vi "6-step.vi"(3 "this":i32, 4 "button":i32, 5 "shift in":bool, 6 "settings in":T1={"Auto1"=TRUE, "Auto2"=TRUE, "Rel1"=TRUE, "Rel2"=TRUE, "Filt1"=TRUE, "Filt2"=TRUE, "Rate"=enum."Slow", "Range1"=enum."10mV", "Range2"=enum."100mV", "Filt3"=TRUE, "Filt4"=TRUE, "Rel temp 1"=TRUE, "Analog1"=FALSE, "Analog2"=FALSE, "Analog temp 1"=FALSE, "Digital1"=TRUE, "Digital2"=TRUE, "Digital temp 1 "=TRUE, "Window1"=enum."0,01%", "Window2"=enum."0,01%", "Window temp 1"=enum."0,01%", "RDGS1"="010", "RDGS2"="010", "RDGS temp 1"="010", "Type_type1"=TRUE, "Type_type2"=TRUE, "Type_type temp 1"=TRUE, "LSync"=FALSE, "Unit"=enum."C", "Sens"=TRUE, "Type tcoupl"=enum."J", "Junc"=TRUE, "prevState"=0, "Rel temp 2"=TRUE, "Analog temp 2"=FALSE, "Digital temp 2"=TRUE, "Type_type temp 2"=TRUE, "RDGS temp 2"="010", "Window temp 2"=enum."0,01%", "addres"="0"}) -> (0 "next state":i32, 1 "shift out":bool, 2 "settings out":T1)   [LabVIEW 2017]
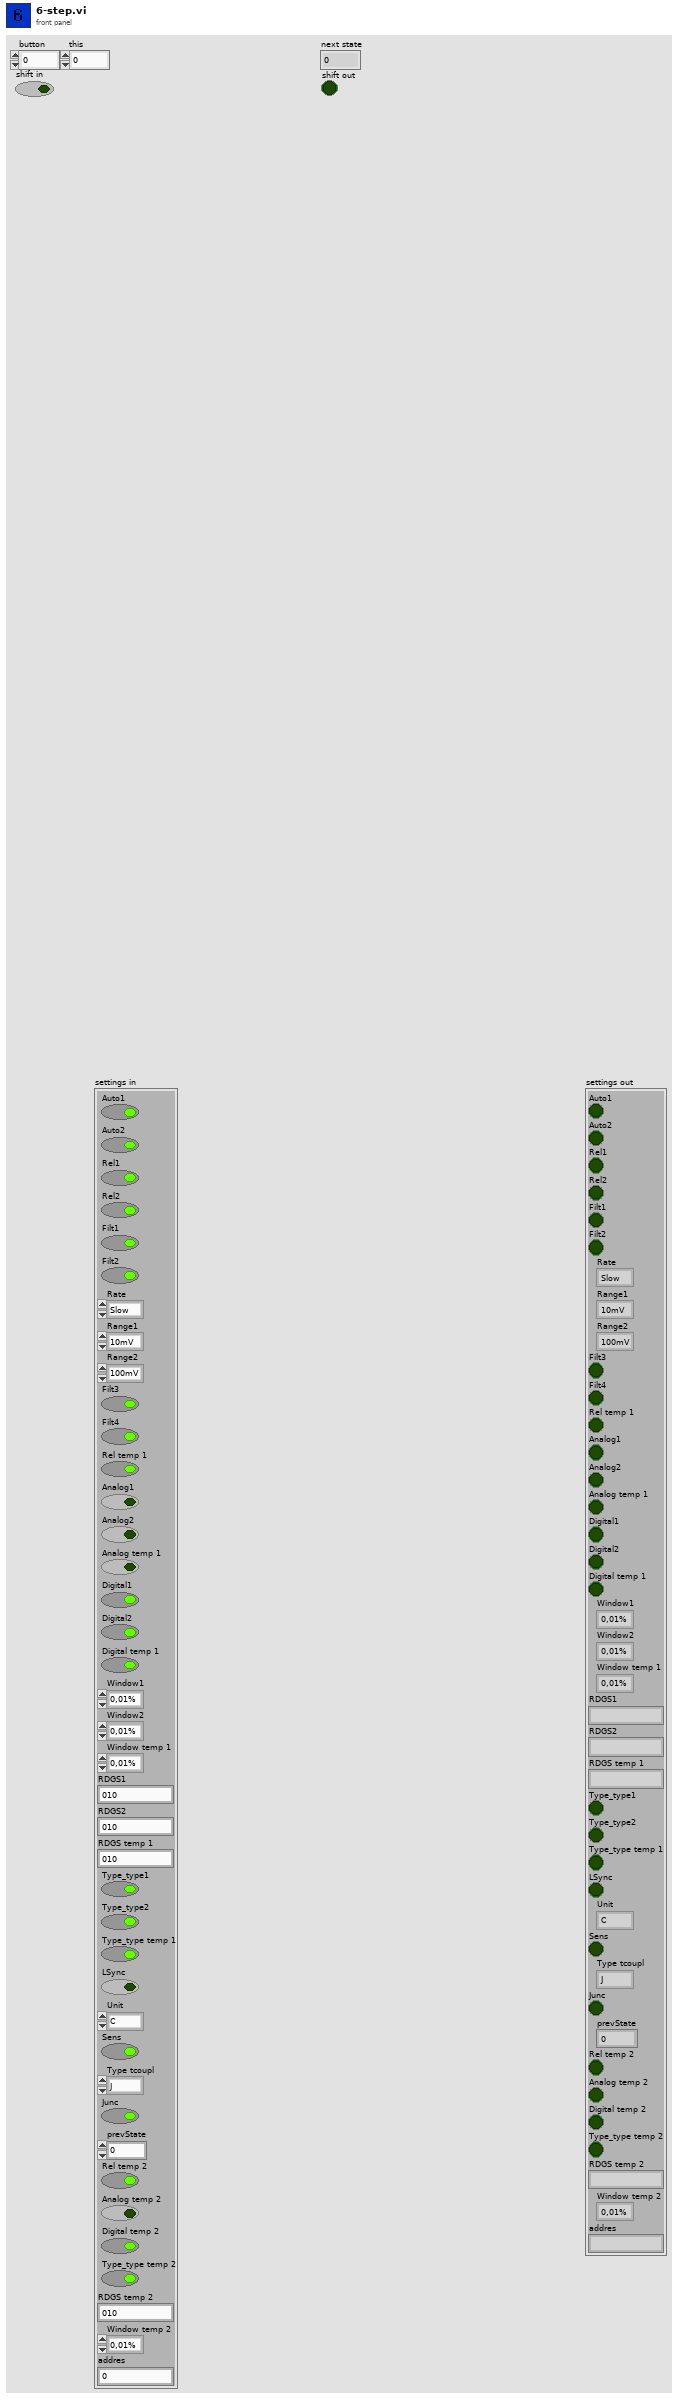
[diagram p1: front panel]
types:
  T1 = cluster{"Auto1":bool, "Auto2":bool, "Rel1":bool, "Rel2":bool, "Filt1":bool, "Filt2":bool, "Rate":enum16{"Slow", "Med", "Fast"}, "Range1":enum16{"10mV", "100mV", "1V", "10V", "100V"}, "Range2":enum16{"100mV", "1V", "10V"}, "Filt3":bool, "Filt4":bool, "Rel temp 1":bool, "Analog1":bool, "Analog2":bool, "Analog temp 1":bool, "Digital1":bool, "Digital2":bool, "Digital temp 1 ":bool, "Window1":enum16{"0,01%", "0,1%", "1%", "10%", "None"}, "Window2":enum16{"0,01%", "0,1%", "1%", "10%", "None"}, "Window temp 1":enum16{"0,01%", "0,1%", "1%", "10%", "None"}, "RDGS1":string, "RDGS2":string, "RDGS temp 1":string, "Type_type1":bool, "Type_type2":bool, "Type_type temp 1":bool, "LSync":bool, "Unit":enum16{"C", "K", "F"}, "Sens":bool, "Type tcoupl":enum16{"J", "K", "T", "E", "R", "S", "B", "N"}, "Junc":bool, "prevState":i32, "Rel temp 2":bool, "Analog temp 2":bool, "Digital temp 2":bool, "Type_type temp 2":bool, "RDGS temp 2":string, "Window temp 2":enum16{"0,01%", "0,1%", "1%", "10%", "None"}, "addres":string}
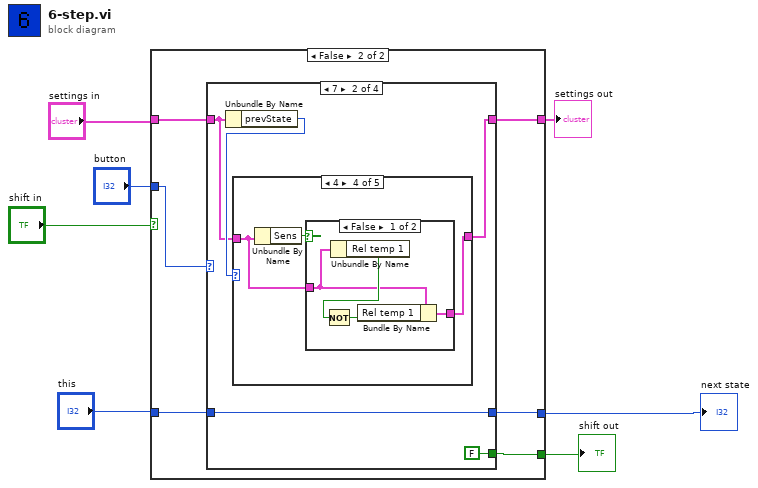
[diagram p0: block diagram]
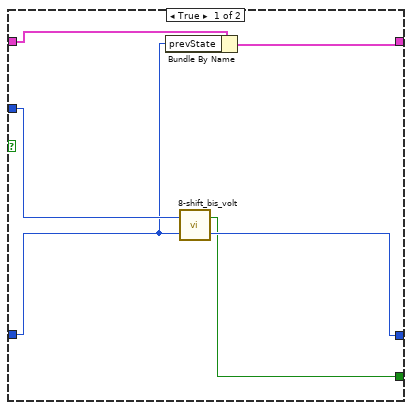
[diagram p2: hidden frame]
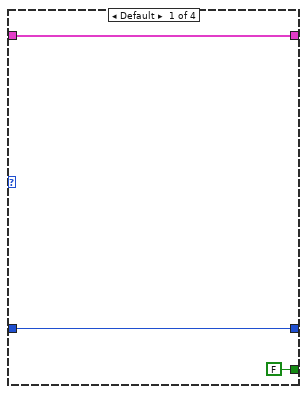
[diagram p3: hidden frame]
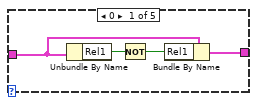
[diagram p4: hidden frame]
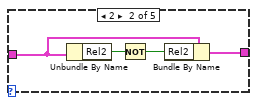
[diagram p5: hidden frame]
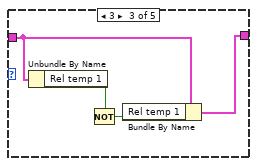
[diagram p6: hidden frame]
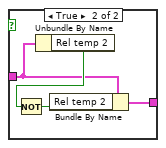
[diagram p7: hidden frame]
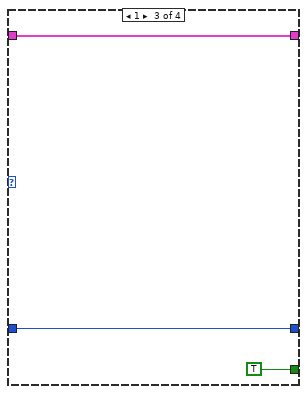
[diagram p9: hidden frame]
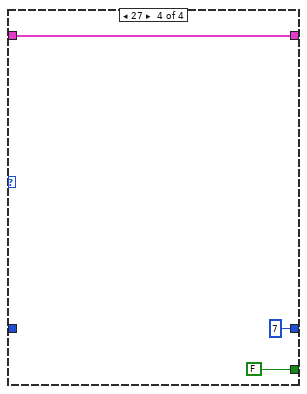
[diagram p10: hidden frame]
diagram:
  n1 = case shown="False" "shift in" {
    tunnel: "button" -> [w13 w19]
    tunnel: [w12 w16] -> w5
    tunnel: "this" -> [w8 w17]
    tunnel: [w11 w18] -> w3
    tunnel: "settings in" -> [w10 w15]
    tunnel: [w9 w14] -> w1
    frame True {
      n2 = Bundle By Name(cluster=w10, "prevState"=w8) -> (w9:T1)
      n3 = call "8-shift_bis_volt.vi"("this"=w8, "button"=w13) -> ("next state"=w12:i32, "shift"=w11:bool)
    }
    frame False {
      n4 = case shown="7" w19 {
        tunnel: [FALSE FALSE TRUE FALSE] -> w18
        tunnel: w17 -> [w22 w27 w53 _]
        tunnel: [w22 w27 w53 7 ("this")] -> w16
        tunnel: [w20 w23 w52 w56] -> w14
        tunnel: w15 -> [w20 w24 w52 w56]
        frame Default {
        }
        frame 7 {
          n5 = Unbundle By Name(w24) -> ("prevState"=w25:i32)
          n6 = case shown="4" w25 {
            tunnel: w24 -> [w29 w33 w37 w41 w51]
            tunnel: [w28 w32 w36 w40 w51] -> w23
            frame 0 {
              n7 = Unbundle By Name(w29) -> ("Rel1"=w31:bool)
              n8 = Not(x=w31) -> (.not. x?=w30:bool)
              n9 = Bundle By Name(cluster=w29, "Rel1"=w30) -> (w28:T1)
            }
            frame 2 {
              n10 = Unbundle By Name(w33) -> ("Rel2"=w35:bool)
              n11 = Not(x=w35) -> (.not. x?=w34:bool)
              n12 = Bundle By Name(cluster=w33, "Rel2"=w34) -> (w32:T1)
            }
            frame 3 {
              n13 = Unbundle By Name(w37) -> ("Rel temp 1"=w39:bool)
              n14 = Not(x=w39) -> (.not. x?=w38:bool)
              n15 = Bundle By Name(cluster=w37, "Rel temp 1"=w38) -> (w36:T1)
            }
            frame 4 {
              n16 = Unbundle By Name(w41) -> ("Sens"=w42:bool)
              n17 = case shown="False" w42 {
                tunnel: w41 -> [w44 w48]
                tunnel: [w43 w47] -> w40
                frame False {
                  n18 = Unbundle By Name(w44) -> ("Rel temp 1"=w46:bool)
                  n19 = Not(x=w46) -> (.not. x?=w45:bool)
                  n20 = Bundle By Name(cluster=w44, "Rel temp 1"=w45) -> (w43:T1)
                }
                frame True {
                  n21 = Unbundle By Name(w48) -> ("Rel temp 2"=w50:bool)
                  n22 = Not(x=w50) -> (.not. x?=w49:bool)
                  n23 = Bundle By Name(cluster=w48, "Rel temp 2"=w49) -> (w47:T1)
                }
              }
            }
            frame Default {
            }
          }
        }
        frame 1 {
        }
        frame 27 {
        }
      }
    }
  }
  "next state" <- w5
  "shift out" <- w3
  "settings out" <- w1
